vi "NormalizeExtension.vi"(10 "Extension":string, 11 "Path in":path) -> (3 "Path out":path)   [LabVIEW 2020]
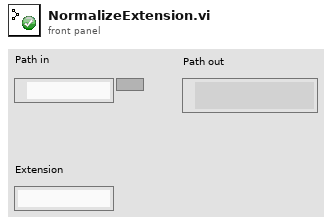
[diagram p1: front panel]
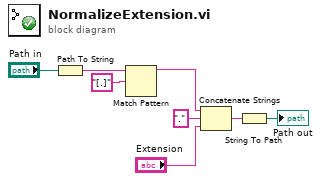
[diagram p0: block diagram]
diagram:
  n1 = Path To String(path="Path in") -> (string=w7:string)
  n2 = Match Pattern(string=w7, regular expression="[.]") -> (before substring=w5:string)  [unwired: 1 in, 3 out]
  n3 = Concatenate Strings(w5, "." ("string"), "Extension") -> (w2:string)
  n4 = String To Path(string=w2) -> (path=→"Path out":path)
